vi "subsystem_logEvent_RejectedCommand.vi"(8 "error in (no error)":errorcluster, 10 "logevent_RejectedCommand in":T1, 11 "ProgrammaticInitialization in":refnum<class "ProgrammaticInitialization.lvclass">) -> (0 "error out":errorcluster, 2 "logevent_RejectedCommand":T1, 3 "ProgrammaticInitialization out":refnum<class "ProgrammaticInitialization.lvclass">)   [LabVIEW 2016, in "ProgrammaticInitialization.lvclass"]
uses:
  ProgrammaticInitialization.lvclass
  ts_sallv_sedspectrometer/DataTypes/logevent_RejectedCommand.ctl
  ts_sallv_sedspectrometer/SALLV_sedSpectrometer.lvlib
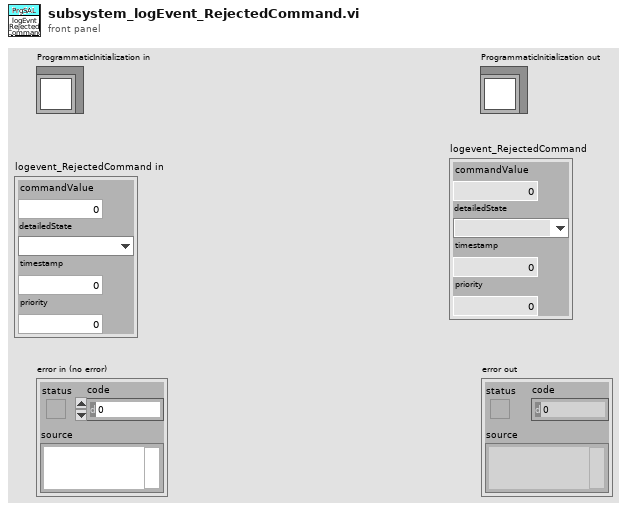
[diagram p1: front panel]
types:
  T1 = typedef "SALLV_sedSpectrometer.lvlib/logevent_RejectedCommand.ctl" = cluster{"commandValue":u16, "detailedState":enum16{"", "DisabledState", "EnabledState", "FaultState", "OfflineState", "StandbyState"}, "timestamp":dbl, "priority":i32}
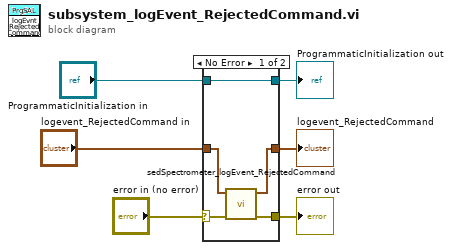
[diagram p0: block diagram]
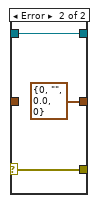
[diagram p2: hidden frame]
diagram:
  n1 = case shown="No Error" "error in (no error)" {
    selector: "error in (no error)" -> [w10 w14]
    tunnel: [w9 w14] -> w5
    tunnel: [w11 w13] -> w3
    tunnel: "ProgrammaticInitialization in" -> [w11 w13]
    tunnel: [w8 T1 {"commandValue"=0, "detailedState"=enum."", "timestamp"=0.0, "priority"=0} ("logevent_RejectedCommand_Ctl out")] -> w2
    tunnel: "logevent_RejectedCommand in" -> [w7 _]
    frame No Error {
      n2 = call "sedSpectrometer_logEvent_RejectedCommand.vi"("error in (no error)"=w10, "logevent_RejectedCommand_Ctl"=w7) -> ("error out"=w9:errorcluster, "logevent_RejectedCommand_Ctl out"=w8:T1)  [unwired: 7 in, 1 out]
    }
    frame Error {
    }
  }
  "error out" <- w5
  "ProgrammaticInitialization out" <- w3
  "logevent_RejectedCommand" <- w2
